vi "Logging.vi"() -> ()   [LabVIEW 2017]
panel:
  out "refnum out":refnum<file>
  in  "refnum in":refnum<file>
  out "Error Out":errorcluster
  in  "Error In":errorcluster
  in  "Battery Number":string
  in  "Date and Time":string
  in  "Match Number":dbl
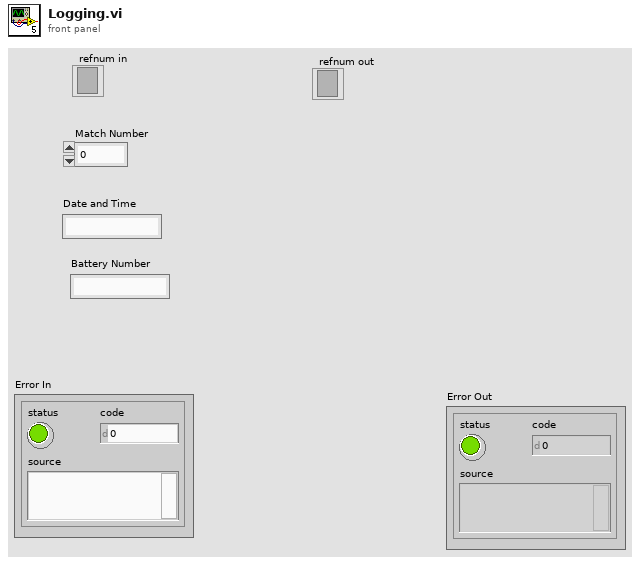
[diagram p1: front panel]
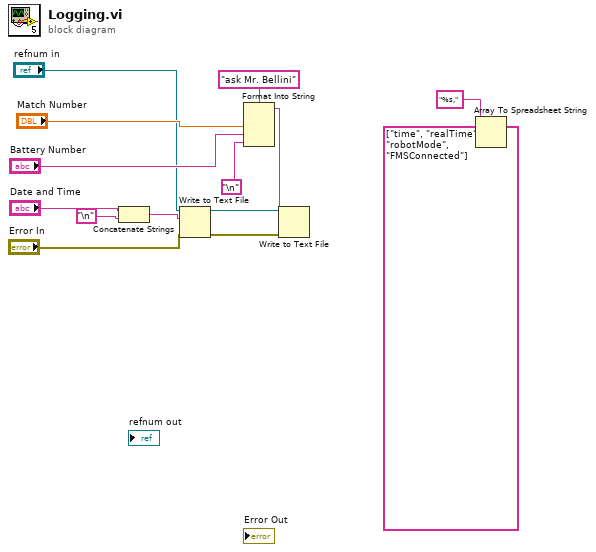
[diagram p0: block diagram]
diagram:
  (unwired) string[] ["time", "realTime", "robotMode", "FMSConnected"]
  n1 = Concatenate Strings("Date and Time", "\n") -> (w7:string)
  n2 = Write to Text File(file (use dialog)="refnum in", text=w7, error in="Error In") -> (refnum out=w5:refnum<file>, error out=w3:errorcluster)  [unwired: 1 in, 1 out]
  n3 = Format Into String(format string="ask Mr. Bellini", "Match Number", "Battery Number", "\n") -> (resulting string=w4:string)  [unwired: 2 in, 1 out]
  n4 = Write to Text File(file (use dialog)=w5, text=w4, error in=w3) -> ()  [unwired: 1 in, 3 out]
  n5 = Array To Spreadsheet String(3:"%s," ("format string")) -> ()  [unwired: 2 in, 1 out]
